vi "Create Response-JSONtext.vi"(6 "id":string, 8 "error in (no error)":errorcluster, 10 "result":variant) -> (0 "error out":errorcluster, 2 "{JSON}":string)   [LabVIEW 2019, in "JSON-RPC.lvclass"]
uses:
  JSON-RPC.lvclass
  8b9e59fa-9ebd-4504-a939-6047597c77d3.vi
  <vilib>/JDP Science/JSONtext/support/Format JSON Object.vi
  <vilib>/JDP Science/JSONtext/Variant to JSON Text.vi
  <vilib>/JDP Science/JSONtext/LVClass Serializer/JSONtext LVClass Serializer.lvclass
  31d5db40-9dcb-43d1-a6f6-9a2e0a5d4432.vi
  <vilib>/JDP Science/JSONtext/JSONtext.lvlib
  c6edfa98-d038-4790-952c-164baa6befaa.vi
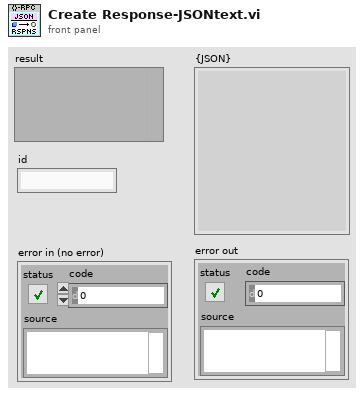
[diagram p1: front panel]
types:
  T1 = cluster{"jsonrpc":string, "result":string, "id":string}
  T2 = typedef "JSON-RPC.lvclass/Error--Cluster.ctl" = cluster{"code":i32, "message":string}
  T3 = cluster{"jsonrpc":string, "error":T2, "id":string}
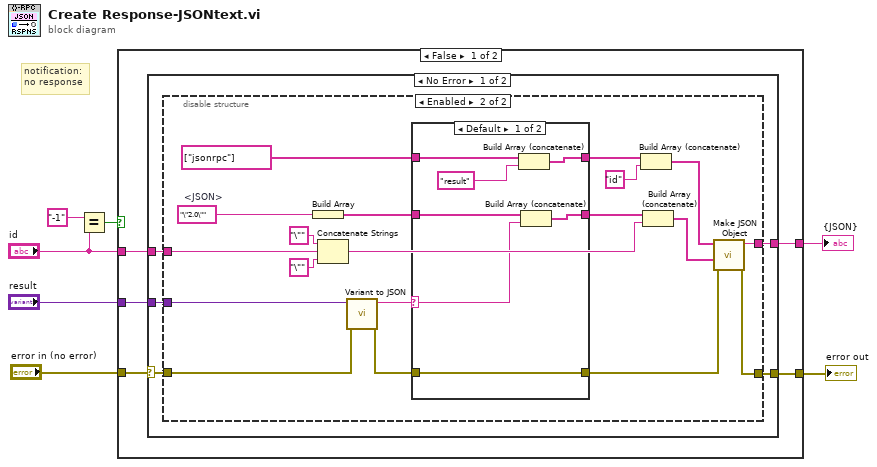
[diagram p0: block diagram]
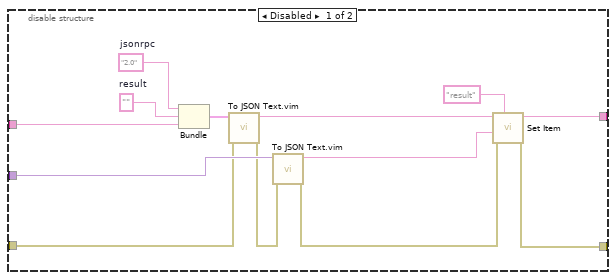
[diagram p2: hidden frame]
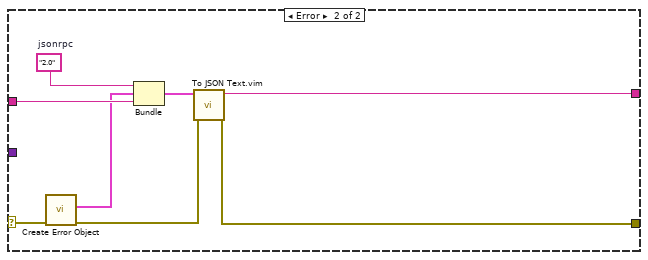
[diagram p4: hidden frame]
diagram:
  # "notification:\nno response"
  n1 = Equal?(x="-1", y="id") -> (x = y?=w1:bool)
  n2 = case shown="False" w1 {
    tunnel: [w12 w68] -> w7
    tunnel: [w11 _] -> w6
    tunnel: "result" -> [w10 _]
    tunnel: "error in (no error)" -> [w9 w68]
    tunnel: "id" -> [w8 _]
    frame False {
      n3 = case shown="No Error" w9 {
        selector: w9 -> [w16 w63]
        tunnel: [w13 w60] -> w12
        tunnel: [w15 w67] -> w11
        tunnel: w8 -> [w14 w66]
        tunnel: w10 -> [w17 _]
        frame No Error {
          n4 = disable-structure shown="Enabled" {
            disable-tunnel: w17 -> [w30 w41]
            disable-tunnel: w16 -> [w26 w36]
            disable-tunnel: [w25 w39] -> w15
            disable-tunnel: w14 -> [w20 w34]
            disable-tunnel: [w19 w40] -> w13
            frame Disabled {
              w18 = ""  # result
              w22 = "2.0"  # jsonrpc
              n5 = Bundle("jsonrpc"=w22, "result"=w18, "id"=w20) -> (w21:T1)  [unwired: 1 in]
              n6 = call "To JSON Text.vim"("error in (no error)"=w26, "Anything"=w21) -> ("error out"=w24:errorcluster, "<JSON>"=w23:string)  [unwired: 8 in]
              n7 = call "To JSON Text.vim"("error in (no error)"=w24, "Anything"=w30) -> ("error out"=w29:errorcluster, "<JSON>"=w28:string)  [unwired: 8 in]
              n8 = call <vilib>:"Set Item.vi"("$Path or Item Name"="result", "error in (no error)"=w29, "JSON to Insert"=w28, "JSON"=w23) -> ("error out"=w19:errorcluster, "<JSON>"=w25:string)  [unwired: 4 in, 1 out]
            }
            frame Enabled {
              w35 = "\"2.0\""  # <JSON>
              n9 = Build Array(w35) -> (w49:string[])
              n10 = Concatenate Strings("\"" ("string"), w34, "\"" ("string")) -> (w31:string)
              n11 = call "Variant to JSON.vi"("error in (no error)"=w36, "variant"=w41) -> ("error out"=w37:errorcluster, "<JSON>"=w38:string)  [unwired: 8 in]
              n12 = case shown="Default" w38 {
                selector: w38 -> [w51 _]
                tunnel: [w52 w59] -> w46
                tunnel: w49 -> [w53 w59]
                tunnel: string[] ["jsonrpc"] -> [w56 w58]
                tunnel: [w54 w58] -> w47
                tunnel: w37 -> [w50 w57]
                tunnel: [w50 w57] -> w43
                frame Default {
                  n13 = Build Array (concatenate)(w56, "result" ("String")) -> (w54:string[])
                  n14 = Build Array (concatenate)(w53, w51) -> (w52:string[])
                }
                frame "null" {
                }
              }
              n15 = Build Array (concatenate)(w47, "id" ("String")) -> (w44:string[])
              n16 = Build Array (concatenate)(w46, w31) -> (w45:string[])
              n17 = call <vilib>:"Make JSON Object.vi"("error in (no error)"=w43, "JSON Items"=w45, "Item Names"=w44) -> ("error out"=w40:errorcluster, "<JSON>"=w39:string)  [unwired: 7 in]
            }
          }
        }
        frame Error {
          w64 = "2.0"  # jsonrpc
          n18 = call "Create Error Object.vi"("error in (no error)"=w63) -> ("error out"=w62:errorcluster, "error"=w61:T2)  [unwired: 9 in]
          n19 = Bundle("jsonrpc"=w64, "error"=w61, "id"=w66) -> (w65:T3)  [unwired: 1 in]
          n20 = call "To JSON Text.vim"("error in (no error)"=w62, "Anything"=w65) -> ("error out"=w60:errorcluster, "<JSON>"=w67:string)  [unwired: 8 in]
        }
      }
    }
    frame True {
    }
  }
  "error out" <- w7
  "{JSON}" <- w6
